vi "UHR-Fleezers Control (host) - 12.1.vi"() -> ()   [LabVIEW 2012] (continued)
        n1597 = feedback #30(refnum<k0> refnum) -> (w2743:refnum<file>)
        n1598 = feedback #31(FALSE ("Save APD Data\nwith Trap Data")) -> (w2751:bool)
        n1599 = feedback #32(refnum<k0> refnum) -> (w2754:refnum<file>)
        n1600 = feedback #33(0) -> (w2770:i32)
        n1601 = feedback #34() -> (w2758:u32)  [unwired: 1 out]
        n1602 = case shown="True" w2765 {
          tunnel: [w2777 1] -> w2766
          tunnel: w2770 -> [w2779 _]
          tunnel: [w2778 w2797] -> w2767
          tunnel: w2768 -> [w2778 _]
          tunnel: w2764 -> [_ w2817]
          tunnel: w2757 -> [_ w2815]
          tunnel: w2759 -> [_ w2818]
          tunnel: [w2776 w2796] -> w2756
          tunnel: w2758 -> [w2776 _]
          tunnel: [w2775 w2794] -> w2753
          tunnel: w2754 -> [w2775 _]
          tunnel: [w2774 w2793] -> w2750
          tunnel: w2751 -> [w2774 _]
          tunnel: "Start Saving" -> [_ w2791]
          tunnel: w2746 -> [_ w2790]
          tunnel: [w2773 w2781] -> w2739
          tunnel: w2743 -> [w2773 _]
          tunnel: [w2772 w2780] -> w2740
          tunnel: w2741 -> [w2772 _]
          frame False {
            n1603 = Increment(x=w2779) -> (x+1=w2777:i32)
          }
          frame True {
            w2787 = FALSE ("Start Saving")
            w2792 = 9.0  # File Version
            w2800 = FALSE ("prepend array or string size? (T)")
            w2798 = T35."big-endian, network order" ("byte order (0:big-endian, network order)")
            n1604 = local read "BD 1 Frequency 1 (MHz)"() -> (w2814:dbl)
            n1605 = local read "BD 2 Frequency 1 (MHz)"() -> (w2813:dbl)
            n1606 = local read "BD 1 Frequency 2 (MHz)"() -> (w2812:dbl)
            n1607 = local read "BD 2 Frequency 2 (MHz)"() -> (w2811:dbl)
            n1608 = local read "BD 1 Frequency 3 (MHz)"() -> (w2810:dbl)
            n1609 = local read "BD 2 Frequency 3 (MHz)"() -> (w2809:dbl)
            n1610 = Array Size(array=w2790) -> (size(s)=w2789:i32)
            n1611 = To Double Precision Float(number=w2789) -> (double precision float=w2788:dbl)
            n1612 = local write "Save Calibration"(w2787) -> ()
            n1613 = local write "Start Saving"(w2787) -> ()
            n1614 = Build Array("Save APD Data\nwith Trap Data", "Save Trap Pos. Data") -> (w2784:bool[])
            n1615 = Boolean Array To Number(Boolean array=w2784) -> (number=w2783:u32)
            n1616 = Build Array(w2814, w2813, w2812, w2811, w2810, w2809) -> (w2808:dbl[])
            n1617 = case shown="1, Default" w2818 {
              tunnel: w2817 -> [w2889 w2909 w2925 w2963]
              tunnel: w2788 -> [w2894 w2916 w2945 w2982]
              tunnel: w2815 -> [w2893 w2915 w2944 w2981]
              tunnel: [w2890 w2911 w2936 w2973] -> w2806
              tunnel: [w2881 "Cal sets to save" w2926 w2964] -> w2796
              tunnel: w2808 -> [w2891 w2912 w2938 w2975]
              tunnel: "Save APD Data\nwith Trap Data" -> [w2888 _ w2922 w2961]
              tunnel: [w2888 w2903 w2922 w2961] -> w2793
              tunnel: w2792 -> [w2884 w2904 w2920 w2959]
              tunnel: w2791 -> [w2883 _ _ _]
              tunnel: [w2874 w2903 w2919 w2949] -> w2780
              tunnel: "Save Trap Pos. Data" -> [w2874 _ w2919 w2949]
              tunnel: w2783 -> [w2873 _ w2918 w2948]
              frame 1, Default {
                # "timeseries"
                n1618 = case shown="True" "Profile" {
                  tunnel: [w2897 w2901] -> w2878
                  tunnel: [w2897 w2900] -> w2877
                  tunnel: [w2897 w2899] -> w2876
                  tunnel: [w2897 w2898] -> w2875
                  frame False {
                    w2897 = 0.0 ("f")
                  }
                  frame True {
                    n1619 = local read "Current Position"() -> (w2902:cluster{dbl, dbl, dbl})
                    n1620 = local read "Y change (mm)"() -> (w2898:dbl)
                    n1621 = Unbundle(w2902) -> (w2901:dbl, w2900:dbl, w2899:dbl)
                  }
                }
                n1622 = local read "Save ave N"() -> (w2896:dbl)
                n1623 = Multiply(x=w2896, y=w2889) -> (x*y=w2895:dbl)
                n1624 = To Double Precision Float(number=w2873) -> (double precision float=w2887:dbl)
                n1625 = Build Array(w2884, w2889, w2895, w2894, w2893, 0.0 ("f")) -> (w2892:dbl[])
                n1626 = Build Array(w2887, w2878, w2877, w2876, w2875) -> (w2885:dbl[])
                n1627 = Select(t=u32 4000000000, s=w2883, f="N sets to save") -> (s? t:f=w2881:u32)
                n1628 = Build Array (concatenate)(w2892, w2891, w2885) -> (w2890:dbl[])
              }
              frame 2 {
                w2906 = 0.0 ("f")
                w2903 = FALSE ("Save APD Data\nwith Trap Data")
                # "calibration"
                n1629 = Boolean To (0,1)(Boolean=w2903) -> (0, 1=w2908:i16)
                n1630 = To Double Precision Float(number=w2908) -> (double precision float=w2907:dbl)
                n1631 = Build Array(w2907, w2906, w2906, w2906, w2906) -> (w2905:dbl[])
                n1632 = Build Array(w2904, w2909, w2909, w2916, w2915, 1.0 ("t")) -> (w2913:dbl[])
                n1633 = Build Array (concatenate)(w2913, w2912, w2905) -> (w2911:dbl[])
                "Calibrating Trap..." <- TRUE ("Calibrating...")
              }
              frame 4 {
                w2923 = 0.0 ("f")
                # "scan dir (x/y = 0/1)"
                # "cycles/step"
                # "n scans (f/b)"
                # "steps"
                # "freq. range"
                # "AOD raster scan"
                n1634 = local read "Number of F/B Scans (AOD)"() -> (w2930:u16)
                n1635 = local read "Cycles/step (AOD)"() -> (w2932:u64)
                n1636 = local read "Scan Range (MHz)"() -> (w2935:dbl)
                n1637 = local read "Scan steps (AOD)"() -> (w2934:u64)
                n1638 = local read "Scan BD"() -> (w2942:bool)
                n1639 = local read "Save ave N"() -> (w2947:dbl)
                n1640 = Boolean To (0,1)(Boolean=w2942) -> (0, 1=w2941:i16)
                n1641 = To Double Precision Float(number=w2930) -> (double precision float=w2929:dbl)
                n1642 = To Double Precision Float(number=w2934) -> (double precision float=w2933:dbl)
                n1643 = To Double Precision Float(number=w2932) -> (double precision float=w2931:dbl)
                n1644 = To Double Precision Float(number=w2941) -> (double precision float=w2940:dbl)
                n1645 = Multiply(x=w2947, y=w2925) -> (x*y=w2946:dbl)
                n1646 = To Double Precision Float(number=w2918) -> (double precision float=w2924:dbl)
                n1647 = Build Array(w2924, w2923, w2923, w2923, w2923) -> (w2921:dbl[])
                n1648 = local read "N sets should be saved"() -> (w2927:dbl)
                n1649 = Build Array(w2940, w2935, w2933, w2931, w2929) -> (w2937:dbl[])
                n1650 = Build Array(w2920, w2925, w2946, w2945, w2944, 2.0 ("t")) -> (w2939:dbl[])
                n1651 = Round Toward +Infinity(x=w2927) -> (ceil(x): smallest int >= x=w2928:dbl)
                n1652 = Build Array (concatenate)(w2939, w2938, w2921, w2937) -> (w2936:dbl[])
                n1653 = To Unsigned Long Integer(number=w2928) -> (unsigned 32bit integer=w2926:u32)
              }
              frame 8 {
                w2956 = 0.0 ("f")
                # "MCL raster scan"
                n1654 = local read "Number of scans (MCL)"() -> (w2951:u64)
                n1655 = local read "Scan lines (y)"() -> (w2950:u64)
                n1656 = local read "2D or 1D Scan"() -> (w2953:bool)
                n1657 = local read "Scan Range (V)\n(of steps)"() -> (w2972:dbl)
                n1658 = local read "Fast Scan Dir"() -> (w2979:bool)
                n1659 = local read "Cycles/step (MCL)"() -> (w2969:u64)
                n1660 = local read "Scan steps (MCL)"() -> (w2971:u64)
                n1661 = Select(t=w2950, s=w2953, f=w2951) -> (s? t:f=w2952:u64)
                n1662 = Boolean To (0,1)(Boolean=w2953) -> (0, 1=w2955:i16)
                n1663 = local read "Save ave N"() -> (w2984:dbl)
                n1664 = local read "Initial X"() -> (w2958:dbl)
                n1665 = local read "Initial Y"() -> (w2957:dbl)
                n1666 = To Double Precision Float(number=w2955) -> (double precision float=w2954:dbl)
                n1667 = Boolean To (0,1)(Boolean=w2979) -> (0, 1=w2978:i16)
                n1668 = To Double Precision Float(number=w2952) -> (double precision float=w2967:dbl)
                n1669 = To Double Precision Float(number=w2971) -> (double precision float=w2970:dbl)
                n1670 = To Double Precision Float(number=w2969) -> (double precision float=w2968:dbl)
                n1671 = To Double Precision Float(number=w2978) -> (double precision float=w2977:dbl)
                n1672 = Multiply(x=w2984, y=w2963) -> (x*y=w2983:dbl)
                n1673 = To Double Precision Float(number=w2948) -> (double precision float=w2962:dbl)
                n1674 = local read "N sets should be saved (MCL)"() -> (w2965:dbl)
                n1675 = Build Array(w2962, w2954, w2956, w2956, w2956) -> (w2960:dbl[])
                n1676 = Build Array(w2977, w2972, w2970, w2968, w2967, w2958, w2957) -> (w2974:dbl[])
                n1677 = Build Array(w2959, w2963, w2983, w2982, w2981, 3.0 ("t")) -> (w2976:dbl[])
                n1678 = Round Toward +Infinity(x=w2965) -> (ceil(x): smallest int >= x=w2966:dbl)
                n1679 = Build Array (concatenate)(w2976, w2975, w2960, w2974) -> (w2973:dbl[])
                n1680 = To Unsigned Long Integer(number=w2966) -> (unsigned 32bit integer=w2964:u32)
              }
            }
            n1681 = local read "Index"() -> (w2823:dbl)
            n1682 = call "Create new save file.vi"("Insert"="", "Ext"=".dat", "Index In"=w2823) -> ("Path Out"=w2782:path, "Index Out"=w2795:dbl)
            n1683 = local write "Save file name"(w2782) -> ()
            n1684 = local write "Index"(w2795) -> ()
            n1685 = local write "Save index"(w2795) -> ()
            n1686 = Array Size(array=w2806) -> (size(s)=w2807:i32)
            n1687 = Open/Create/Replace File(file path (use dialog)=w2782, operation (0:open)=T34."create", access (0:read/write)=enum16{"read/write", "read-only", "write-only"}."write-only") -> (refnum out=w2820:refnum<file>)  [unwired: 1 in, 4 out]
            n1688 = local write "Saving..."(TRUE ("Saving...")) -> ()
            n1689 = To Double Precision Float(number=w2807) -> (double precision float=w2805:dbl)
            n1690 = String Length(string="Comment (data description)") -> (length=w2803:i32)
            n1691 = To Double Precision Float(number=w2803) -> (double precision float=w2802:dbl)
            n1692 = Deny Access(7:w2820) -> (3:w2819:refnum<file>)  [unwired: 1 in, 2 out]
            n1693 = Build Array (concatenate)(w2805, w2806, w2802) -> (w2804:dbl[])
            n1694 = case "If fluorescence data to be saved" shown="True" w2793 {
              tunnel: w2782 -> [_ w2872]
              tunnel: [refnum<k0> refnum w2852] -> w2794
              frame False {
              }
              frame True {
                w2851 = 0.0
                n1695 = local read "APD Integration Time (s)"() -> (w2857:dbl)
                n1696 = local read "N APD Samp/step"() -> (w2850:dbl)
                n1697 = Path To String(path=w2872) -> (string=w2871:string)
                n1698 = String Length(string=w2871) -> (length=w2870:i32)
                n1699 = Subtract(x=w2870, y=4) -> (x-y=w2868:i32)
                n1700 = String Subset(string=w2871, length (rest)=w2868) -> (substring=w2867:string)  [unwired: 1 out]
                n1701 = Build Array(w2857, w2850, w2851, w2851, w2851, w2851, w2851, w2851) -> (w2854:dbl[])
                n1702 = Concatenate Strings(w2867, "_fl.dat" ("string")) -> (w2865:string)
                n1703 = Array Size(array=w2854) -> (size(s)=w2856:i32)
                n1704 = String To Path(string=w2865) -> (path=w2861:path)
                n1705 = Open/Create/Replace File(file path (use dialog)=w2861, operation (0:open)=T34."create", access (0:read/write)=enum16{"read/write", "read-only", "write-only"}."write-only") -> (refnum out=w2862:refnum<file>)  [unwired: 1 in, 4 out]
                n1706 = Deny Access(7:w2862) -> (3:w2858:refnum<file>)  [unwired: 1 in, 2 out]
                n1707 = To Double Precision Float(number=w2856) -> (double precision float=w2855:dbl)
                n1708 = Build Array (concatenate)(w2855, w2854) -> (w2853:dbl[])
                n1709 = Write to Binary File(file (use dialog)=w2858, data=w2853, 5:FALSE ("prepend array or string size? (T)"), 9:T35."big-endian, network order" ("byte order (0:big-endian, network order)")) -> (refnum out=w2852:refnum<file>)  [unwired: 1 in, 3 out]
              }
            }
            n1710 = case shown="True" w2780 {
              tunnel: w2782 -> [_ w2834]
              tunnel: [refnum<k0> refnum w2833] -> w2781
              frame False {
              }
              frame True {
                w2829 = 0.0 ("element")
                n1711 = Path To String(path=w2834) -> (string=w2848:string)
                n1712 = Build Array(w2829, w2829, w2829, w2829, w2829, w2829, w2829, w2829) -> (w2830:dbl[])
                n1713 = String Length(string=w2848) -> (length=w2847:i32)
                n1714 = Subtract(x=w2847, y=4) -> (x-y=w2845:i32)
                n1715 = Array Size(array=w2830) -> (size(s)=w2832:i32)
                n1716 = String Subset(string=w2848, length (rest)=w2845) -> (substring=w2844:string)  [unwired: 1 out]
                n1717 = To Double Precision Float(number=w2832) -> (double precision float=w2831:dbl)
                n1718 = Concatenate Strings(w2844, "_pos.dat" ("string")) -> (w2842:string)
                n1719 = Build Array (concatenate)(w2831, w2830) -> (w2828:dbl[])
                n1720 = String To Path(string=w2842) -> (path=w2838:path)
                n1721 = Open/Create/Replace File(file path (use dialog)=w2838, operation (0:open)=T34."create", access (0:read/write)=enum16{"read/write", "read-only", "write-only"}."write-only") -> (refnum out=w2839:refnum<file>)  [unwired: 1 in, 4 out]
                n1722 = Deny Access(7:w2839) -> (3:w2835:refnum<file>)  [unwired: 1 in, 2 out]
                n1723 = Write to Binary File(file (use dialog)=w2835, data=w2828, 5:FALSE ("prepend array or string size? (T)"), 9:T35."big-endian, network order" ("byte order (0:big-endian, network order)")) -> (refnum out=w2833:refnum<file>)  [unwired: 1 in, 3 out]
              }
            }
            n1724 = Write to Binary File(file (use dialog)=w2819, data=w2804, 5:w2800, 9:w2798) -> (refnum out=w2801:refnum<file>)  [unwired: 1 in, 3 out]
            n1725 = Write to Binary File(file (use dialog)=w2801, data="Comment (data description)", 5:w2800, 9:w2798) -> (refnum out=w2797:refnum<file>)  [unwired: 1 in, 3 out]
          }
        }
        n1726 = feedback-in #28(w2740) -> ()
        n1727 = feedback-in #29(w2767) -> ()
        n1728 = feedback-in #30(w2739) -> ()
        n1729 = feedback-in #31(w2750) -> ()
        n1730 = feedback-in #32(w2753) -> ()
        n1731 = feedback-in #33(w2766) -> ()
        n1732 = feedback-in #34(w2756) -> ()
      }
      frame #1 {
        n1733 = local read "Saving..."() -> (w2998:bool)
        n1734 = case shown="True" w2998 {
          tunnel: w3002 -> [_ w3013]
          tunnel: w3001 -> [_ w3027]
          tunnel: w3000 -> [_ w3023]
          tunnel: w2999 -> [_ w3022]
          tunnel: w2997 -> [_ w3021]
          tunnel: w2996 -> [_ w3016]
          tunnel: w2995 -> [_ w3015]
          tunnel: w2994 -> [_ w3014]
          tunnel: w2993 -> [_ w3012]
          tunnel: w2992 -> [_ w3010]
          tunnel: w2991 -> [_ w3009]
          tunnel: w2990 -> [_ w3008]
          tunnel: w2989 -> [_ w3007]
          tunnel: w2988 -> [_ w3006]
          tunnel: w2987 -> [_ w3005]
          tunnel: w2986 -> [_ w3004]
          tunnel: w2985 -> [_ w3003]
          frame False {
          }
          frame True {
            n1735 = Multiply(x=w3013, y=w3012) -> (x*y=→"Time (s)":dbl)
            n1736 = Less Or Equal?(x=w3013, y=w3021) -> (x <= y?=w3025:bool)
            n1737 = Or(x="Stop Saving", y="Abort save 2") -> (x .or. y?=w3017:bool)
            n1738 = Not(x=w3017) -> (.not. x?=w3026:bool)
            n1739 = And(x=w3025, y=w3026) -> (x .and. y?=w3024:bool)
            n1740 = case shown="True" w3024 {
              tunnel: w3027 -> [w3034 w3109]
              tunnel: [0.0 w3112] -> w3020
              tunnel: w3013 -> [_ w3110]
              tunnel: w3021 -> [_ w3111]
              tunnel: w3023 -> [_ w3106]
              tunnel: w3022 -> [_ _]
              tunnel: w3016 -> [w3032 w3099]
              tunnel: w3015 -> [w3031 w3100]
              tunnel: w3014 -> [_ w3098]
              tunnel: w3010 -> [_ w3097]
              tunnel: w3009 -> [_ w3041]
              tunnel: w3008 -> [_ w3090]
              tunnel: w3007 -> [_ w3068]
              tunnel: w3006 -> [w3028 w3050]
              tunnel: w3005 -> [w3029 w3049]
              tunnel: w3004 -> [_ w3046]
              tunnel: w3003 -> [_ w3044]
              frame False {
                w3030 = FALSE
                n1741 = Close File(refnum=w3034) -> ()  [unwired: 1 in, 2 out]
                n1742 = case shown="True" w3031 {
                  tunnel: w3032 -> [_ w3036]
                  frame False {
                  }
                  frame True {
                    n1743 = Close File(refnum=w3036) -> ()  [unwired: 1 in, 2 out]
                  }
                }
                n1744 = case shown="True" w3028 {
                  tunnel: w3029 -> [_ w3035]
                  frame False {
                  }
                  frame True {
                    n1745 = Close File(refnum=w3035) -> ()  [unwired: 1 in, 2 out]
                  }
                }
                n1746 = local write "Raster Scanning..."(w3030) -> ()
                n1747 = local write "Calibrating Trap..."(w3030) -> ()
                n1748 = call <vilib>:"Beep.vi"() -> ()  [unwired: 3 in, 9 out]
                n1749 = local write "Stop Saving"(w3030) -> ()
                "Saving..." <- w3030
              }
              frame True {
                n1750 = local read "Calibrating Trap..."() -> (w3101:bool)
                n1751 = case "Write fl. data" shown="True" w3100 {
                  tunnel: w3099 -> [_ w3135]
                  tunnel: w3098 -> [_ w3134]
                  frame False {
                  }
                  frame True {
                    n1752 = Write to Binary File(file (use dialog)=w3135, data=w3134, 5:FALSE ("prepend array or string size? (T)"), 9:T35."big-endian, network order" ("byte order (0:big-endian, network order)")) -> ()  [unwired: 1 in, 4 out]
                  }
                }
                n1753 = Greater?(x="Save ave N", y=1.0) -> (0:w3104:bool)
                n1754 = Not(x=w3101) -> (.not. x?=w3103:bool)
                n1755 = And(x=w3103, y=w3104) -> (x .and. y?=w3047:bool)
                n1756 = case shown="True" w3047 {
                  tunnel: w3046 -> [w3115 w3126]
                  tunnel: [w3115 w3118] -> w3045
                  tunnel: "Save ave N" -> [_ w3119]
                  frame False {
                  }
                  frame True {
                    w3116 = 2 ("dimension size")
                    n1757 = Array Size(array=w3126) -> (size(s)=w3120:i32)
                    n1758 = Divide(x=w3120, y=w3116) -> (x/y=w3124:dbl)
                    n1759 = Reshape Array(w3126, w3124, w3116) -> (w3125:u64[][])
                    n1760 = Transpose 2D Array(2D array=w3125) -> (transposed array=w3123:u64[][])
                    n1761 = for {
                      tunnel: w3123 -> [w3128] mode=indexing
                      tunnel: [w3127] -> w3117 mode=indexing
                      tunnel: w3119 -> [w3129]
                      workers-P: _ -> [_]
                      n1762 = call "downsample 1D array - U64.vi"("Ave N"=w3129, "Array In"=w3128) -> ("Array Out"=w3127:u64[])  [unwired: 1 in]
                    }
                    n1763 = Transpose 2D Array(2D array=w3117) -> (transposed array=w3122:u64[][])
                    n1764 = Divide(x=w3120, y=w3119) -> (x/y=w3121:dbl)
                    n1765 = Reshape Array(w3122, w3121) -> (w3118:u64[])
                  }
                }
                n1766 = case shown="True" w3047 {
                  tunnel: w3106 -> [w3138 w3150]
                  tunnel: [w3138 w3142] -> w3102
                  tunnel: "Save ave N" -> [_ w3143]
                  tunnel: w3097 -> [_ w3141]
                  frame False {
                  }
                  frame True {
                    n1767 = Array Size(array=w3150) -> (size(s)=w3144:i32)
                    n1768 = Array Size(array=w3141) -> (size(s)=w3140:i32)
                    n1769 = Divide(x=w3144, y=w3140) -> (x/y=w3148:dbl)
                    n1770 = Reshape Array(w3150, w3148, w3140) -> (w3149:i16[][])
                    n1771 = Transpose 2D Array(2D array=w3149) -> (transposed array=w3147:i16[][])
                    n1772 = for {
                      tunnel: w3147 -> [w3153] mode=indexing
                      tunnel: [w3152] -> w3139 mode=indexing
                      tunnel: w3143 -> [w3151]
                      workers-P: _ -> [_]
                      n1773 = call "downsample 1D array - I16.vi"("Ave N"=w3151, "Array In"=w3153) -> ("Array Out"=w3152:i16[])  [unwired: 1 out]
                    }
                    n1774 = Transpose 2D Array(2D array=w3139) -> (transposed array=w3146:i16[][])
                    n1775 = Divide(x=w3144, y=w3143) -> (x/y=w3145:dbl)
                    n1776 = Reshape Array(w3146, w3145) -> (w3142:i16[])
                  }
                }
                n1777 = Index Array(array=w3068, index=1) -> (element=w3071:waveform(dbl))
                n1778 = Index Array(array=w3068, index=0) -> (element=w3073:waveform(dbl))
                n1779 = Unbundle By Name(w3071) -> ("Y"=w3075:dbl[])
                n1780 = Unbundle By Name(w3073) -> ("Y"=w3083:dbl[])
                n1781 = case "Write trap pos. data" shown="True" w3050 {
                  tunnel: w3049 -> [_ w3131]
                  tunnel: w3045 -> [_ w3130]
                  frame False {
                  }
                  frame True {
                    n1782 = Write to Binary File(file (use dialog)=w3131, data=w3130, 5:FALSE ("prepend array or string size? (T)"), 9:T35."big-endian, network order" ("byte order (0:big-endian, network order)")) -> ()  [unwired: 1 in, 4 out]
                  }
                }
                n1783 = Write to Binary File(file (use dialog)=w3109, data=w3102, 5:FALSE ("prepend array or string size? (T)"), 9:T35."big-endian, network order" ("byte order (0:big-endian, network order)")) -> ()  [unwired: 1 in, 4 out]
                n1784 = feedback #35(w3075) -> (w3077:dbl[])
                n1785 = Build Array (concatenate)(w3077, w3075) -> (w3076:dbl[])
                n1786 = Select(t=w3075, s=w3041, f=w3076) -> (s? t:f=w3061:dbl[])
                n1787 = feedback-in #35(w3061) -> ()
                n1788 = feedback #36(w3083) -> (w3096:dbl[])
                n1789 = Build Array (concatenate)(w3096, w3083) -> (w3095:dbl[])
                n1790 = Select(t=w3083, s=w3041, f=w3095) -> (s? t:f=w3070:dbl[])
                n1791 = feedback-in #36(w3070) -> ()
                n1792 = Divide(x=w3110, y=w3111) -> (x/y=w3113:dbl)
                n1793 = Multiply(x=w3113, y=100.0) -> (x*y=w3112:dbl)
                n1794 = Build Array(w3070, w3061) -> (→"Saved APD":dbl[][])
                n1795 = Array Size(array=w3070) -> (size(s)=w3088:i32)
                n1796 = Unbundle By Name(w3090) -> ("Y"=w3094:dbl[])
                n1797 = Subtract(x=w3088, y="N pts to average") -> (x-y=w3064:i32)
                n1798 = Multiply(x="N pts to average", y=u16 2) -> (x*y=w3065:u16)
                n1799 = Subtract(x=w3088, y=w3065) -> (x-y=w3063:i32)
                n1800 = feedback #37(w3094) -> (w3093:dbl[])
                n1801 = Build Array (concatenate)(w3093, w3094) -> (w3092:dbl[])
                n1802 = Select(t=w3094, s=w3041, f=w3092) -> (s? t:f=w3091:dbl[])
                "Trap Delta Graph" <- w3091
                n1803 = feedback-in #37(w3091) -> ()
                n1804 = Array Subset(array=w3070, index=w3064, length="N pts to average") -> (w3087:dbl[])
                n1805 = Array Subset(array=w3070, index=w3063, length="N pts to average") -> (w3086:dbl[])
                n1806 = Array Subset(array=w3061, index=w3064, length="N pts to average") -> (w3067:dbl[])
                n1807 = Array Subset(array=w3061, index=w3063, length="N pts to average") -> (w3066:dbl[])
                n1808 = Index Array(array=w3044, index=0) -> (element=w3042:waveform(dbl))
                n1809 = call-poly <vilib>:"Mean.vi"("X"=w3087) -> ("mean"=w3085:dbl)  [unwired: 1 out]
                n1810 = call-poly <vilib>:"Mean.vi"("X"=w3067) -> ("mean"=w3060:dbl)  [unwired: 1 out]
                n1811 = call-poly <vilib>:"Mean.vi"("X"=w3086) -> ("mean"=w3084:dbl)  [unwired: 1 out]
                n1812 = call-poly <vilib>:"Mean.vi"("X"=w3066) -> ("mean"=w3059:dbl)  [unwired: 1 out]
                n1813 = Unbundle By Name(w3042) -> ("Y"=w3039:dbl[])
                n1814 = Subtract(x=w3060, y=w3059) -> (x-y=w3051:dbl)
                "Delta Fl. 2" <- w3051
                n1815 = Subtract(x=w3085, y=w3084) -> (x-y=w3082:dbl)
                "Delta Fl. 1" <- w3082
                n1816 = Initialize Array(w3082, 1 ("dimension size")) -> (w3079:dbl[])
                n1817 = Initialize Array(w3051, 1 ("dimension size")) -> (w3056:dbl[])
                n1818 = feedback #38(w3079) -> (w3080:dbl[])
                n1819 = Build Array (concatenate)(w3080, w3079) -> (w3078:dbl[])
                n1820 = feedback #39(w3056) -> (w3057:dbl[])
                n1821 = Build Array (concatenate)(w3057, w3056) -> (w3055:dbl[])
                n1822 = feedback #40(w3039) -> (w3038:dbl[])
                n1823 = Build Array (concatenate)(w3038, w3039) -> (w3040:dbl[])
                n1824 = Select(t=w3039, s=w3041, f=w3040) -> (s? t:f=w3037:dbl[])
                "Saved trap pos" <- w3037
                n1825 = feedback-in #40(w3037) -> ()
                n1826 = Select(t=w3079, s=w3041, f=w3078) -> (s? t:f=w3054:dbl[])
                n1827 = feedback-in #38(w3054) -> ()
                n1828 = Select(t=w3056, s=w3041, f=w3055) -> (s? t:f=w3053:dbl[])
                n1829 = feedback-in #39(w3053) -> ()
                n1830 = Build Array(w3054, w3053) -> (→"Save APD Deriv":dbl[][])
              }
            }
            "Progress" <- w3020
            "Progress 2" <- w3020
          }
        }
      }
    }
    n1831 = local read "wait to reset values"() -> (w1749:bool)
    n1832 = Not(x=w1747) -> (.not. x?=w1750:bool)
    n1833 = And(x=w1750, y=w1749) -> (x .and. y?=w1751:bool)
    n1834 = case "Part of MCL raster scanning: returns to initial positions after scan done" shown="True" w1751 {
      tunnel: w1472 -> [w2560 w2567]
      tunnel: [w2560 w2566] -> w1753
      tunnel: w1471 -> [w2559 w2565]
      tunnel: [w2559 w2564] -> w1748
      frame False {
      }
      frame True {
        w2575 = 10.0 ("y")
        w2574 = 32767.0 ("y")
        # "to return scan values\nafter a synchronous \nAOM scan"
        n1835 = local read "AO2"() -> (w2568:dbl)
        n1836 = local read "AO1"() -> (w2569:dbl)
        n1837 = local write "wait to reset values"(FALSE ("wait to reset values")) -> ()
        n1838 = Multiply(x=w2569, y=w2574) -> (x*y=w2571:dbl)
        n1839 = Multiply(x=w2568, y=w2574) -> (x*y=w2573:dbl)
        n1840 = Divide(x=w2571, y=w2575) -> (x/y=w2570:dbl)
        n1841 = Divide(x=w2573, y=w2575) -> (x/y=w2572:dbl)
        n1842 = To Word Integer(number=w2570) -> (16bit integer=w2576:i16)
        n1843 = To Word Integer(number=w2572) -> (16bit integer=w2577:i16)
        n1844 = local read "Total Counts (ticks)"() -> (w2561:u32)
        n1845 = xnode "Read/Write Control"("FPGA VI Reference In"=w2567, "error in"=w2565, "AO1"=w2576, "AO2"=w2577, "MCL count"=w2561) -> ("FPGA VI Reference Out"=w2566:T18, "error out"=w2564:errorcluster)
        n1846 = local read "Scan Range (V)\n(of steps)"() -> (w2562:dbl)
        n1847 = property on="Scan Range (V)\n(of steps)" class="DigNum (strict)"("Val(Sgnl)"=w2562) -> ()  [unwired: 2 in, 2 out]
      }
    }
    n1848 = node-c288() -> ()  [unwired: 2 out]
  }
  n1849 = timed-loop "Control parameters (event loop)" {
    tunnel: w28 -> [w3162]
    shift-right: [w3161] -> _
    shift-left: errorcluster {"status"=FALSE, "code"=0, "source"=""} ("error out") -> [w3160]
    tunnel: [w3159] -> _
    timing: w116 -> [_]
    timing-out: [_] -> w115
    tunnel: w88 -> [w3158]
    tunnel: w32 -> [w3157]
    tunnel: w31 -> [w3156]
    tunnel: w30 -> [w3155]
    tunnel: w29 -> [w3154]
    stop <- w3159 stop-if-true
    n1850 = node-c288() -> ()  [unwired: 2 out]
    n1851 = event shown="[45] \"Sample Channel Flow\": Value Change" {
      selector: _ -> [_ _ _ _ _ _ _ _ _ _ _ _ _ _ _ _ _ _ _ _ _ _ _ _ _ _ _ _ _ _ _ _ _ _ _ _ _ _ _ _ _ _ _ _ _ _ _ _ _ _ _ _ _ _ _ _ _ _ _ _ _ _ _ _ _ _ _ _ _ _ _ _ _ _ _ _]
      dyn-events: _ -> [_ _ _ _ _ _ _ _ _ _ _ _ _ _ _ _ _ _ _ _ _ _ _ _ _ _ _ _ _ _ _ _ _ _ _ _ _ _ _ _ _ _ _ _ _ _ _ _ _ _ _ _ _ _ _ _ _ _ _ _ _ _ _ _ _ _ _ _ _ _ _ _ _ _ _ _]
      timeout: _ -> [_ _ _ _ _ _ _ _ _ _ _ _ _ _ _ _ _ _ _ _ _ _ _ _ _ _ _ _ _ _ _ _ _ _ _ _ _ _ _ _ _ _ _ _ _ _ _ _ _ _ _ _ _ _ _ _ _ _ _ _ _ _ _ _ _ _ _ _ _ _ _ _ _ _ _ _]
      tunnel: w3162 -> [w3203 _ _ _ w3241 _ w3263 _ _ _ _ w3329 _ _ w3372 w3378 w3385 w3390 w3426 w3447 w3454 _ w3466 w3470 w3481 w3492 w3503 w3514 w3525 w3536 w3563 w3657 w3662 w3700 _ w3735 w3739 w3750 w3754 w3758 _ w3766 _ _ _ _ _ _ _ _ _ _ _ _ _ _ _ _ _ w4144 _ w4161 _ w4168 w4186 _ w4193 w4201 w4216 w4232 w4238 _ w4247 _ w4266 _]
      tunnel: [w3202 _ _ _ w3231 _ w3262 _ _ w3294 _ w3308 _ _ w3371 w3374 w3384 w3387 w3425 w3445 w3453 _ w3464 _ w3475 w3486 w3497 w3508 w3519 w3530 w3561 w3655 w3660 w3698 _ w3733 w3737 w3740 w3752 w3756 _ w3764 _ _ _ _ _ _ _ _ _ _ _ _ _ _ _ _ _ w4142 _ _ _ _ w4183 _ _ _ _ _ _ _ _ _ _ _] -> w3161
      tunnel: w3160 -> [w3201 _ _ _ w3240 _ w3261 _ _ w3294 _ w3328 _ _ w3370 w3373 w3383 w3386 w3424 w3446 w3452 _ w3465 w3469 w3480 w3491 w3502 w3513 w3524 w3535 w3562 w3656 w3661 w3699 _ w3734 w3738 w3749 w3753 w3757 _ w3765 _ _ _ _ _ _ _ _ _ _ _ _ _ _ _ _ _ w4143 _ w4160 _ w4167 w4185 _ w4192 w4200 w4215 w4231 w4237 _ w4246 _ w4265 _]
      tunnel: [_ _ _ _ _ _ _ _ _ w3293 _ _ _ _ _ _ _ _ _ _ _ _ _ _ _ _ _ _ _ _ _ _ _ _ _ _ _ _ _ _ _ _ _ _ _ _ _ _ _ _ _ _ _ _ _ _ _ _ _ _ _ _ _ _ _ _ _ _ _ _ _ _ _ _ _ _] -> w3159
      tunnel: [_ _ _ _ _ _ _ "Round T1 X" _ _ _ _ _ _ _ _ _ _ _ _ _ _ _ _ _ _ _ _ _ _ _ _ _ _ _ _ _ _ _ _ _ _ _ _ _ _ _ _ _ _ _ _ _ _ _ _ _ _ _ _ _ _ _ _ _ _ _ _ _ _ _ _ _ _ _ _] -> _
      tunnel: [_ _ _ "Adjust Scale\nto Mean" _ _ _ _ _ _ _ _ _ _ _ _ _ _ _ _ _ _ "Test ttrig" _ _ _ _ _ _ _ _ _ _ _ _ _ _ _ _ _ _ _ _ _ _ _ _ _ _ "Flush Sample" "Flush Pump 3" "Flush Pump 1" "Clear Volume" _ _ _ _ _ _ _ _ _ _ _ _ _ _ _ _ _ _ _ _ _ _ _] -> _
      tunnel: [_ _ _ _ _ _ _ _ "Round T2 X" _ "Delayed Interlace Start" _ _ _ _ _ _ _ _ _ _ _ _ _ _ _ _ _ _ _ _ _ _ _ _ _ _ _ _ _ _ _ _ _ _ _ _ _ _ _ _ _ _ _ _ _ _ _ _ _ _ _ _ _ _ _ _ _ _ _ _ _ _ _ _ _] -> _
      tunnel: w3158 -> [_ _ _ _ _ _ _ _ _ _ _ _ _ _ _ _ _ _ _ _ _ _ _ _ _ _ _ _ _ _ _ _ _ _ _ _ _ _ _ _ _ _ _ _ _ w3923 w3930 w3937 w3942 w3951 _ _ w4057 _ _ _ _ _ _ _ _ _ _ _ _ _ _ _ _ _ _ _ _ _ _ _]
      tunnel: w3157 -> [_ _ _ _ _ _ _ _ _ _ _ _ _ _ _ _ _ _ _ _ _ _ _ _ _ _ _ _ _ _ _ _ _ _ _ _ _ _ _ _ _ _ _ w3840 _ _ _ _ _ _ w3995 _ _ w4063 _ w4072 _ w4086 _ _ _ _ _ _ _ _ _ _ _ _ _ _ _ _ _ _]
      tunnel: w3156 -> [_ _ _ _ _ _ _ _ _ _ _ _ _ _ _ _ _ _ _ _ _ _ _ _ _ _ _ _ _ _ _ _ _ _ _ _ _ _ _ _ _ _ _ _ _ _ _ _ _ _ _ _ _ _ _ _ _ _ _ _ _ _ _ _ _ _ _ _ _ _ _ _ _ _ _ _]
      tunnel: w3155 -> [_ _ _ _ _ _ _ _ _ _ _ _ _ _ _ _ _ _ _ _ _ _ _ _ _ _ _ _ _ _ _ _ _ _ _ _ _ _ _ _ _ _ w3777 _ _ _ _ _ _ _ _ w4025 _ _ w4068 _ w4079 _ w4111 _ _ _ _ _ _ _ _ _ _ _ _ _ _ _ _ _]
      tunnel: w3154 -> [_ _ _ _ _ _ _ _ _ _ _ _ _ _ _ _ _ _ _ _ _ _ _ _ _ _ _ _ _ _ _ _ _ _ _ _ _ _ _ _ _ _ _ _ _ _ _ _ _ _ _ _ _ _ _ _ _ _ _ _ _ _ _ _ _ _ _ _ _ _ _ _ _ _ _ _]
      event "AI Count (ticks)", "Sets to FIFO (Traps)", "Save ave N", "FPGA Ave.", "# Samples/channel", "N sets to save": Value Change {
        # "So that if 'Save ave N' is updated, the AOD scanning code updates too."
        n1852 = event-data() -> ()  [unwired: 6 out]
        n1853 = local read "AI Count (ticks)"() -> (w3184:u32)
        n1854 = Unbundle By Name("Sets to FIFO (Traps)") -> ("Set 1"=w3167:bool, "Set 2"=w3166:bool, "Set 3"=w3165:bool)
        n1855 = Boolean To (0,1)(Boolean="Sets to FIFO (Traps)") -> (0, 1=w3193:cluster{"Set 1":i16, "Set 2":i16, "Set 3":i16})
        n1856 = xnode "Read/Write Control"("FPGA VI Reference In"=w3203, "error in"=w3201, "ai count"=w3184, "Set 1"=w3167, "Set 2"=w3166, "Set 3"=w3165, "N of AI1 Int Acq Sets"="N Acq Sets (Traps + Fl.)") -> ("error out"=w3202:errorcluster)  [unwired: 1 out]
        n1857 = Cluster To Array(cluster=w3193) -> (array=w3192:i16[])
        n1858 = To Unsigned Long Integer(number=w3192) -> (unsigned 32bit integer=w3173:u32[])
        n1859 = local read "Scan steps (AOD)"() -> (w3194:u64)
        n1860 = Multiply(x=w3184, y="N Acq Sets (Traps + Fl.)") -> (x*y=w3182:u32)
        n1861 = Divide(x=40000000.0, y=w3184) -> (x/y=w3176:dbl)
        "AI rate (Hz)" <- w3176
        "Ave. Rate (Hz)" <- w3176
        n1862 = Add Array Elements(numeric array=w3173) -> (sum=w3185:u32)
        "Trap Sets" <- w3185
        n1863 = Reciprocal(x=w3176) -> (1/x=→"Ave. Period (s)":dbl)
        n1864 = property on="Scan steps (AOD)" class="DigNum (strict)"("Val(Sgnl)"=w3194) -> ()  [unwired: 2 in, 2 out]
        n1865 = Divide(x=w3176, y="N Acq Sets (Traps + Fl.)") -> (x/y=w3198:dbl)
        "Data Rate (Hz)" <- w3198
        n1866 = Reciprocal(x=w3198) -> (1/x=→"Data Period (s)":dbl)
        n1867 = local read "Save ave N"() -> (w3197:dbl)
        n1868 = Divide(x=w3198, y=w3197) -> (x/y=w3196:dbl)
        "Save Data Rate (Hz)" <- w3196
        n1869 = Reciprocal(x=w3196) -> (1/x=→"Save Data Period (s)":dbl)
        n1870 = Multiply(x=w3182, y="# Samples/trap") -> (x*y=w3180:u32)
        "Counts/DMA" <- w3180
        n1871 = property on="Trap Disp. Downsample" class="DigNum (strict)"("Maximum"="# Samples/trap") -> ()  [unwired: 2 in, 2 out]
        n1872 = Multiply(x=w3185, y="# Samples/trap") -> (x*y=w3174:u32)
        "# Samples/channel" <- w3174
        n1873 = Multiply(x=w3174, y=u32 8) -> (x*y=→"Trap AI Elements/DMA read":u32)
        n1874 = local read "APD Int. Count"() -> (w3181:u32)
        n1875 = Multiply(x=w3174, y=u32 3) -> (x*y=→"Trap Pos Elements/DMA read":u32)
        n1876 = Divide(x=w3180, y=w3181) -> (x/y=w3171:dbl)
        "APD Samples/FIFO Acq." <- w3171
        n1877 = Divide(x=w3180, y=40000000.0) -> (x/y=w3178:dbl)
        "DMA Update Period (s)" <- w3178
        n1878 = Multiply(x=2.0, y=w3171) -> (x*y=→"APD Elements/DMA read":dbl)
        n1879 = property on="APD Disp. Downsample" class="DigNum (strict)"("Maximum"=w3171) -> ()  [unwired: 2 in, 2 out]
        n1880 = local read "N sets to save"() -> (w3190:u32)
        n1881 = Multiply(x=w3178, y=w3190) -> (x*y=→"Total Time (s)":dbl)
        "FPGA Averaging" <- FALSE ("FPGA Averaging")
      }
      event "Remove Offset": Value Change {
        n1882 = event-data() -> ()  [unwired: 7 out]
        n1883 = local write "Remove Offset"(FALSE ("Remove Offset")) -> ()
        n1884 = local read "Bead Mean (nm)"() -> (w3205:dbl)
        n1885 = local read "Offset (nm)"() -> (w3206:dbl)
        n1886 = Add(x=w3205, y=w3206) -> (x+y=w3204:dbl)
        n1887 = local write "Offset (nm)"(w3204) -> ()
        n1888 = disable-structure shown="Disabled" {
          frame Disabled {
            n1889 = local read "Bead Mean (nm)"() -> (w3211:dbl)
            n1890 = Add(y=w3211) -> (x=w3210:dbl, x+y=w3209:dbl)
            n1891 = Subtract(x=w3211, y=w3210) -> (x-y=w3208:dbl)
            n1892 = property on="Bead Separation" class="WFChart (strict)"("YScale.Minimum"=w3208) -> ()  [unwired: 2 in, 2 out]
            n1893 = property on="Bead Separation" class="WFChart (strict)"("YScale.Maximum"=w3209) -> ()  [unwired: 2 in, 2 out]
          }
          frame Enabled {
          }
        }
      }
      event "Detector Type": Value Change {
        n1894 = event-data() -> ()  [unwired: 7 out]
        n1895 = local read "AI labels"() -> (w3212:string[])
        n1896 = property on="High Res. Display" class="Ring (strict)"("Strings []"=w3212) -> ()  [unwired: 2 in, 2 out]
        n1897 = Build Array (concatenate)(w3212, "none") -> (w3213:string[])
        n1898 = property on="FFT 1 Choice 1" class="Ring (strict)"("Strings []"=w3213) -> ()  [unwired: 2 in, 2 out]
        n1899 = property on="FFT 1 Choice 2" class="Ring (strict)"("Strings []"=w3213) -> ()  [unwired: 2 in, 2 out]
        n1900 = property on="FFT 2 Choice 1" class="Ring (strict)"("Strings []"=w3213) -> ()  [unwired: 2 in, 2 out]
        n1901 = property on="FFT 2 Choice 2" class="Ring (strict)"("Strings []"=w3213) -> ()  [unwired: 2 in, 2 out]
        n1902 = Bundle("APD 1", "APD 2") -> (w3216:cluster{string, string})  [unwired: 1 out]
        n1903 = Cluster To Array(cluster=w3216) -> (array=w3214:string[])
        n1904 = Build Array (concatenate)(w3214, w3213) -> (w3218:string[])
        n1905 = Array Size(array=w3218) -> (size(s)=w3219:i32)
        n1906 = property on="Signals to Plot" class="LstBox (strict)"("Item Names"=w3218) -> ()  [unwired: 2 in, 2 out]
        n1907 = property on="Signals to Plot" class="LstBox (strict)"("Number of Rows"=w3219) -> ()  [unwired: 2 in, 2 out]
        n1908 = property on="All Signals" class="WFChart (strict)"("LegNumRows"=w3219) -> ()  [unwired: 2 in, 2 out]
      }
      event "Adjust Scale\nto Mean": Value Change {
        n1909 = event-data() -> ()  [unwired: 7 out]
        n1910 = local read "APD 1 Rate (Hz)"() -> (w3228:dbl)
        n1911 = Multiply(x=1000.0, y="Above (kHz)") -> (x*y=w3226:dbl)
        n1912 = Multiply(x=1000.0, y="Below (kHz)") -> (x*y=w3224:dbl)
        n1913 = Add(x=w3226, y=w3228) -> (x+y=w3221:dbl)
        n1914 = Subtract(x=w3228, y=w3224) -> (x-y=w3222:dbl)
        n1915 = property on="APD Chart" class="WFChart (strict)"("YScale.Minimum"=w3222) -> ()  [unwired: 2 in, 2 out]
        n1916 = property on="APD Chart" class="WFChart (strict)"("YScale.Maximum"=w3221) -> ()  [unwired: 2 in, 2 out]
      }
      event "Phase adj. (AI1)", "+ phase (AI1)", "- phase (AI1)": Value Change {
        n1917 = event-data() -> ()  [unwired: 7 out]
        n1918 = Negate(x="Phase adj. (AI1)") -> (-x=w3238:i16)
        n1919 = Select(t=w3238, s="- phase (AI1)", f="Phase adj. (AI1)") -> (s? t:f=w3237:i16)
        n1920 = xnode "Read/Write Control"("FPGA VI Reference In"=w3241, "error in"=w3240, "Phase count adjustment"=w3237) -> ("FPGA VI Reference Out"=w3236:T18, "error out"=w3235:errorcluster)
        n1921 = Or(x="- phase (AI1)", y="+ phase (AI1)") -> (x .or. y?=w3232:bool)
        n1922 = xnode "Read/Write Control"("FPGA VI Reference In"=w3236, "error in"=w3235, "+ phase"=w3232) -> ("error out"=w3231:errorcluster)  [unwired: 1 out]
      }
      event "Signals to Plot": Double Click {
        w3244 = u32 9868950 ("Color Box")
        n1923 = event-data() -> ("Row"=w3246:i32)  [unwired: 9 out]
        n1924 = property on="All Signals" class="WFChart (strict)"("Active Plot"=w3246) -> (error out=w3257:errorcluster)  [unwired: 2 in, 1 out]
        n1925 = property on="All Signals" class="WFChart (strict)" props=["Plot", "Visible?", "Plot", "Plot Color"](error in=w3257) -> (error out=w3256:errorcluster, "Plot.Visible?"=w3255:bool)  [unwired: 1 in, 2 out]
        n1926 = Select(t=FALSE ("Plot.Visible"), s=w3255, f=TRUE ("Plot.Visible")) -> (s? t:f=w3250:bool)
        n1927 = property on="All Signals" class="WFChart (strict)"(error in=w3256, "Plot.Visible?"=w3250) -> (error out=w3252:errorcluster)  [unwired: 1 in, 1 out]
        n1928 = property on="All Signals" class="WFChart (strict)"(error in=w3252) -> (error out=w3247:errorcluster, "Plot.Plot Color"=w3251:u32)  [unwired: 1 in, 1 out]
        n1929 = property on="Signals to Plot" class="LstBox (strict)"(error in=w3247, "Active Row"=w3246) -> (error out=w3245:errorcluster)  [unwired: 1 in, 1 out]
        n1930 = Select(t=w3251, s=w3250, f=u32 0) -> (s? t:f=w3248:u32)
        n1931 = property on="Signals to Plot" class="LstBox (strict)"(error in=w3245, "CellFontColor"=w3248, "SelColor"=w3244, "CellBG"=w3244, "CellFontSize"=u32 20 ("Active Row:Cell Font:Size"), "CellFontBold"=TRUE ("Active Row:Cell Font:Bold")) -> ()  [unwired: 1 in, 2 out]
      }
      event "BD 1 Frequency 1 (MHz)", "BD 1 Frequency 2 (MHz)", "BD 1 Frequency 3 (MHz)", "BD 2 Frequency 1 (MHz)", "BD 2 Frequency 2 (MHz)", "BD 2 Frequency 3 (MHz)", "Trap Delta (MHz)": Value Change {
        n1932 = event-data() -> ("CtlRef"=w3260:refnum<vi>)  [unwired: 6 out]
        n1933 = control-ref of="Trap Delta (MHz)"() -> (w3259:refnum<vi>)
        n1934 = Equal?(x=w3259, y=w3260) -> (x = y?=w3258:bool)
        n1935 = case shown="False" "Oscillate Set 1" {
          tunnel: w3263 -> [w3283 _]
          tunnel: [w3282 w3286] -> w3262
          tunnel: w3261 -> [w3281 w3286]
          tunnel: w3258 -> [w3266 _]
          frame False {
            n1936 = local read "BD 1 Frequency 2 (MHz)"() -> (w3270:dbl)
            n1937 = local read "BD 1 Frequency 1 (MHz)"() -> (w3268:dbl)
            n1938 = Subtract(x=w3270, y="Trap Delta (MHz)") -> (x-y=w3267:dbl)
            n1939 = Select(t=w3267, s=w3266, f=w3268) -> (s? t:f=w3265:dbl)
            n1940 = local read "Y RF Frequency Limits (MHz)"() -> (w3271:T15)
            n1941 = local read "X RF Frequency Limits (MHz)"() -> (w3272:T15)
            n1942 = local read "BD 1 Frequency 3 (MHz)"() -> (w3284:dbl)
            n1943 = local write "BD 1 Frequency 1 (MHz)"(w3265) -> ()
            n1944 = local read "BD 2 Frequency 1 (MHz)"() -> (w3275:dbl)
            n1945 = local read "BD 2 Frequency 2 (MHz)"() -> (w3274:dbl)
            n1946 = local read "BD 2 Frequency 3 (MHz)"() -> (w3285:dbl)
            n1947 = call "set RF board frequency - interlace.vi"("Board 2 Frequency Limits"=w3271, "Board 1 Frequency Limits"=w3272, "error in"=w3281, "FPGA VI Reference In"=w3283, "Board 2 Frequency 3 (MHz)"=w3285, "Board 1 Frequency 3 (MHz)"=w3284, "Board 2 Frequency 2 (MHz)"=w3274, "Board 2 Frequency 1 (MHz)"=w3275, "Board 1 Frequency 2 (MHz)"=w3270, "Board 1 Frequency 1  (MHz)"=w3265) -> ("error out"=w3282:errorcluster)  [unwired: 1 out]
            n1948 = Subtract(x=w3275, y=w3274) -> (x-y=w3279:dbl)
            n1949 = Subtract(x=w3265, y=w3270) -> (x-y=w3280:dbl)
            n1950 = Square(x=w3279) -> (x^2=w3277:dbl)
            n1951 = Square(x=w3280) -> (x^2=w3278:dbl)
            n1952 = Add(x=w3278, y=w3277) -> (x+y=w3276:dbl)
            n1953 = Square Root(x=w3276) -> (sqrt(x)=w3273:dbl)
            n1954 = local write "Trap Delta (MHz)"(w3273) -> ()
            n1955 = property on="Initial delta (MHz)" class="DigNum (strict)"("Val(Sgnl)"=w3273) -> ()  [unwired: 2 in, 2 out]
          }
          frame True {
          }
        }
      }
      event "Round T1 X": Value Change {
        n1956 = event-data() -> ()  [unwired: 7 out]
        n1957 = local read "BD 1 Frequency 1 (MHz)"() -> (w3289:dbl)
        n1958 = Round To Nearest(number=w3289) -> (nearest integer value=w3288:dbl)
        n1959 = property on="BD 1 Frequency 1 (MHz)" class="DigNum (strict)"("Val(Sgnl)"=w3288) -> ()  [unwired: 2 in, 2 out]
      }
      event "Round T2 X": Value Change {
        n1960 = event-data() -> ()  [unwired: 7 out]
        n1961 = local read "BD 1 Frequency 2 (MHz)"() -> (w3291:dbl)
        n1962 = Round To Nearest(number=w3291) -> (nearest integer value=w3290:dbl)
        n1963 = property on="BD 1 Frequency 2 (MHz)" class="DigNum (strict)"("Val(Sgnl)"=w3290) -> ()  [unwired: 2 in, 2 out]
      }
      event "Stop All": Value Change {
        n1964 = event-data() -> ()  [unwired: 7 out]
        n1965 = local read "Stop All"() -> (w3293:bool)
      }
      event "Delayed Interlace Start": Value Change {
        n1966 = event-data() -> ()  [unwired: 7 out]
        n1967 = flat-sequence {
          frame #0 {
            n1968 = Multiply(x="Delay to Interlace (s)", y=1000.0) -> (x*y=w3296:dbl)
            n1969 = Wait (ms)(milliseconds to wait=w3296) -> ()  [unwired: 1 out]
          }
          frame #1 {
            n1970 = property on="Green laser mode" class="RadioBtnsControl (strict)"("Val(Sgnl)"=enum32{"Laser ON", "Laser OFF", "Interlace"}."Interlace" ("Value (Signaling)")) -> ()  [unwired: 2 in, 2 out]
          }
        }
      }
      event "BD 1 Amplitude 1 (%)", "BD 1 Amplitude 2 (%)", "BD 1 Amplitude 3 (%)", "BD 2 Amplitude 1 (%)", "BD 2 Amplitude 2 (%)", "BD 2 Amplitude 3 (%)", "Trap 1 ON", "Trap 2 ON", "Trap 3 ON", "Feedback On/Off", "All FB On/Off": Value Change {
        w3320 = i16 1 ("f")
        n1971 = event-data() -> ()  [unwired: 7 out]
        n1972 = local write "Trap 1 (ON/OFF)"("Trap 1 ON") -> ()
        n1973 = local write "Trap 2 (ON/OFF)"("Trap 2 ON") -> ()
        n1974 = Boolean To (0,1)(Boolean="Trap 3 ON") -> (0, 1=w3321:i16)
        n1975 = Boolean To (0,1)(Boolean="Trap 1 ON") -> (0, 1=w3322:i16)
        n1976 = Boolean To (0,1)(Boolean="Trap 2 ON") -> (0, 1=w3323:i16)
        n1977 = Select(t=w3323, s="Trap ON/OFF X or Y Amp?", f=w3320) -> (s? t:f=w3318:i16)
        n1978 = Select(t=w3322, s="Trap ON/OFF X or Y Amp?", f=w3320) -> (s? t:f=w3319:i16)
        n1979 = Select(t=w3321, s="Trap ON/OFF X or Y Amp?", f=w3320) -> (s? t:f=w3317:i16)
        n1980 = Select(t=w3320, s="Trap ON/OFF X or Y Amp?", f=w3323) -> (s? t:f=w3315:i16)
        n1981 = Select(t=w3320, s="Trap ON/OFF X or Y Amp?", f=w3322) -> (s? t:f=w3316:i16)
        n1982 = Select(t=w3320, s="Trap ON/OFF X or Y Amp?", f=w3321) -> (s? t:f=w3314:i16)
        n1983 = And(x="All FB On/Off", y="Feedback On/Off") -> (x .and. y?=w3312:cluster{"Set 1":bool, "Set 2":bool})
        n1984 = local read "BD 1 Amplitude 1 (%)"() -> (w3332:dbl)
        n1985 = local read "BD 1 Amplitude 2 (%)"() -> (w3331:dbl)
        n1986 = local read "BD 1 Amplitude 3 (%)"() -> (w3330:dbl)
        n1987 = Unbundle By Name(w3312) -> ("Set 1"=w3307:bool, "Set 2"=w3304:bool)
        n1988 = local read "Y RF Amplitude Limits (%)"() -> (w3300:T15)
        n1989 = local read "X RF Amplitude Limits (%)"() -> (w3301:T15)
        n1990 = local read "BD 2 Amplitude 1 (%)"() -> (w3333:dbl)
        n1991 = local read "BD 2 Amplitude 2 (%)"() -> (w3334:dbl)
        n1992 = local read "BD 2 Amplitude 3 (%)"() -> (w3335:dbl)
        n1993 = And(x="Trap 2 ON", y=w3304) -> (x .and. y?=w3302:bool)
        n1994 = And(x="Trap 1 ON", y=w3307) -> (x .and. y?=w3305:bool)
        n1995 = Multiply(x=w3319, y=w3332) -> (x*y=w3327:dbl)
        n1996 = Multiply(x=w3331, y=w3318) -> (x*y=w3325:dbl)
        n1997 = Multiply(x=w3330, y=w3317) -> (x*y=w3326:dbl)
        n1998 = Multiply(x=w3333, y=w3316) -> (x*y=w3336:dbl)
        n1999 = Multiply(x=w3334, y=w3315) -> (x*y=w3337:dbl)
        n2000 = Multiply(x=w3335, y=w3314) -> (x*y=w3338:dbl)
        n2001 = call "set RF board amplitude - interlace.vi"("Board 2 Amplitude Limits"=w3300, "Board 1 Amplitude Limits"=w3301, "error in"=w3328, "FPGA VI Reference In"=w3329, "Board 2 Amplitude 3 (%)"=w3338, "Board 1 Amplitude 3 (%)"=w3326, "Board 2 Amplitude 2 (%)"=w3337, "Board 2 Amplitude 1 (%)"=w3336, "Board 1 Amplitude 2 (%)"=w3325, "Board 1 Amplitude 1 (%)"=w3327) -> ("error out"=w3309:errorcluster, "FPGA VI Reference Out"=w3310:T18)
        n2002 = xnode "Read/Write Control"("FPGA VI Reference In"=w3310, "error in"=w3309, "FB On/Off Set 1"=w3305, "FB On/Off Set 2"=w3302) -> ("error out"=w3308:errorcluster)  [unwired: 1 out]
      }
      event "Load parameters": Value Change {
        n2003 = event-data() -> ()  [unwired: 7 out]
        n2004 = property on="Saved AOD Raster Scan Parameter Sets" class="Arr (strict)"() -> ("Index Values"=w3349:u32[])  [unwired: 2 in, 2 out]
        n2005 = Index Array(array=w3349, index=0) -> (element=w3346:u32)
        n2006 = local write "Load parameters"(FALSE ("Load parameters")) -> ()
        n2007 = Index Array(array="Saved AOD Raster Scan Parameter Sets", index=w3346) -> (element=w3345:T42)
        n2008 = Unbundle By Name(w3345) -> ("Scan Range AOD (nm) 2"=w3344:dbl, "Step Size AOD (nm) 2"=w3343:dbl, "Scan Speed AOD (nm/s) 2"=w3342:dbl, "Number of scans (AOD) 2"=w3341:u16)
        n2009 = flat-sequence {
          tunnel: w3344 -> [w3352]
          tunnel: w3343 -> [w3351]
          tunnel: w3342 -> [w3350]
          tunnel: w3341 -> [w3353]
          frame #0 {
            n2010 = local write "Scan Speed (nm/s)"(w3350) -> ()
            n2011 = local write "Scan Range (nm)"(w3352) -> ()
            n2012 = local write "Step Size (nm)"(w3351) -> ()
          }
          frame #1 {
            n2013 = property on="Number of F/B Scans (AOD)" class="DigNum (strict)"("Val(Sgnl)"=w3353) -> ()  [unwired: 2 in, 2 out]
          }
        }
      }
      event "Trap 1 (ON/OFF)", "Trap 2 (ON/OFF)": Value Change {
        n2014 = event-data() -> ()  [unwired: 7 out]
        n2015 = property on="Trap 2 ON" class="Bool (strict)"("Val(Sgnl)"="Trap 2 (ON/OFF)") -> ()  [unwired: 2 in, 2 out]
        n2016 = property on="Trap 1 ON" class="Bool (strict)"("Val(Sgnl)"="Trap 1 (ON/OFF)") -> ()  [unwired: 2 in, 2 out]
      }
      event "DIO count 1 (ticks)", "DIO count 2 (ticks)", "DIO count 3 (ticks)", "Interlace", "Number Interlace Sets", "Not-Interlacing Set": Value Change {
        n2017 = event-data() -> ()  [unwired: 7 out]
        n2018 = local read "DIO count 3 (ticks)"() -> (w3366:u32)
        n2019 = local read "DIO count 1 (ticks)"() -> (w3368:u32)
        n2020 = local read "DIO count 2 (ticks)"() -> (w3367:u32)
        n2021 = To Unsigned Byte Integer(number="Not-Interlacing Set") -> (unsigned 8bit integer=w3357:u8)
        n2022 = Add(x=w3357, y=u8 1) -> (x+y=w3361:u8)
        n2023 = xnode "Read/Write Control"("FPGA VI Reference In"=w3372, "error in"=w3370, "DIO count 1 (ticks)"=w3368, "DIO count 2 (ticks)"=w3367, "DIO count 3 (ticks)"=w3366, "Interlace ON/OFF"="Interlace", "Number Interlace Cycles"="Number Interlace Sets", "Interlace Off Parameters"=w3361) -> ("error out"=w3371:errorcluster)  [unwired: 1 out]
        n2024 = Build Array(w3368, w3367, w3366) -> (w3359:u32[])
        n2025 = Split 1D Array(array=w3359, index="Number Interlace Sets") -> (first subarray=w3369:u32[])  [unwired: 1 out]
        n2026 = Index Array(array=w3359, index=w3357) -> (element=w3358:u32)
        n2027 = Add Array Elements(numeric array=w3369) -> (sum=w3363:u32)
        n2028 = Select(t=w3363, s="Interlace", f=w3358) -> (s? t:f=→"Total Counts (ticks)":u32)
      }
      event "Reset Feedback": Value Change {
        n2029 = event-data() -> ()  [unwired: 7 out]
        n2030 = Unbundle By Name("Reset Feedback") -> ("Set 1"=w3376:bool, "Set 2"=w3375:bool)
        n2031 = xnode "Read/Write Control"("FPGA VI Reference In"=w3378, "error in"=w3373, "FB Reset Set 1"=w3376, "FB Reset Set 2"=w3375) -> ("error out"=w3374:errorcluster)  [unwired: 1 out]
      }
      event "Trap Intensity PID Gains": Value Change {
        n2032 = event-data() -> ()  [unwired: 7 out]
        n2033 = Unbundle By Name("Trap Intensity PID Gains") -> ("proportional gain (Kc)"=w3381:i16, "integral gain (Kc*Ts/Ti)"=w3380:i16, "derivative gain (Kc*Td/Ts)"=w3379:i16)
        n2034 = xnode "Read/Write Control"("FPGA VI Reference In"=w3385, "error in"=w3383, "P1"=w3381, "I1"=w3380, "D1"=w3379) -> ("error out"=w3384:errorcluster)  [unwired: 1 out]
      }
      event "AI2 to Setpoint", "Setpoints (V)": Value Change {
        n2035 = event-data() -> ()  [unwired: 7 out]
        n2036 = xnode "Read/Write Control"("FPGA VI Reference In"=w3390, "error in"=w3386) -> ("FPGA VI Reference Out"=w3389:T18, "error out"=w3388:errorcluster, "AI2 Y Sum Set 1"=w3397:i16, "AI2 Y Sum Set 2"=w3396:i16)
        n2037 = Cluster To Array(cluster="AI2 to Setpoint") -> (array=w3400:bool[])
        n2038 = local read "AI2 (V)"() -> (w3398:cluster{"Set 1":dbl, "Set 2":dbl})
        n2039 = Or Array Elements(Boolean array=w3400) -> (logical OR=w3401:bool)
        n2040 = Bundle By Name(cluster=w3398, "Set 1"=w3397, "Set 2"=w3396) -> (w3395:cluster{"Set 1":dbl, "Set 2":dbl})
        n2041 = Divide(x=w3395, y=3276.7) -> (x/y=w3394:cluster{"Set 1":dbl, "Set 2":dbl})
        "AI2 (V)" <- w3394
        n2042 = case shown="True" w3401 {
          tunnel: [w3404 w3421] -> w3393
          tunnel: "AI2 to Setpoint" -> [_ w3417]
